vi "disc_PI.vi"(0 "y_ref":dbl, 1 "PISettiings":cluster{"Kp":dbl, "Ti":dbl}, 2 "Ts":dbl, 3 "manual":u16, 4 "u_man":dbl, 5 "y":dbl) -> (14 "u_k":dbl)   [LabVIEW 2019]
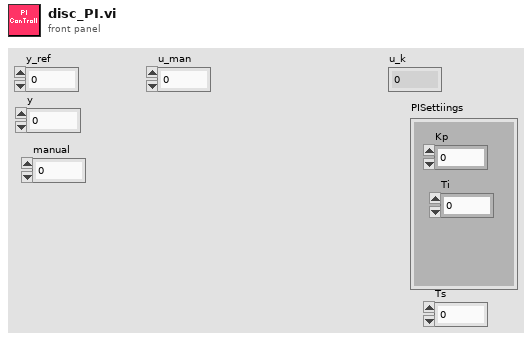
[diagram p1: front panel]
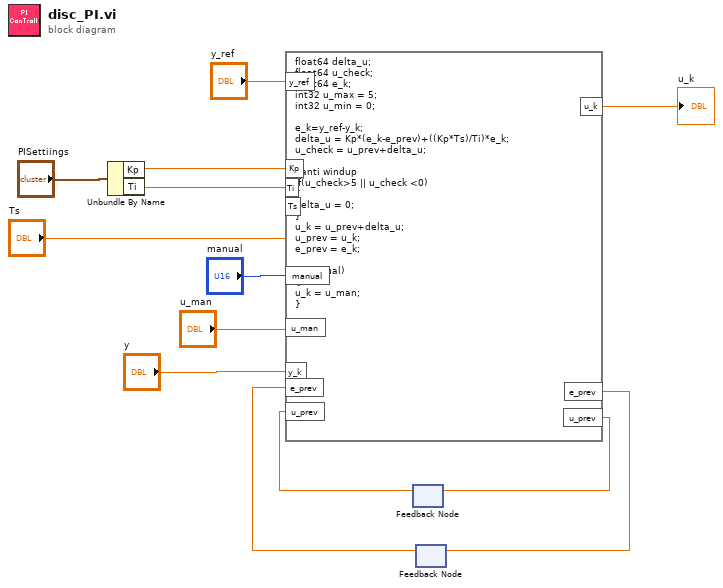
[diagram p0: block diagram]
diagram:
  n1 = Unbundle By Name("PISettiings") -> ("Kp"=w6:dbl, "Ti"=w5:dbl)
  n2 = feedback #1() -> (w8:dbl)  [unwired: 1 in]
  n3 = feedback #2() -> (w2:dbl)  [unwired: 1 in]
  n4 = formula code="float64 delta_u;\nfloat64 u_check;\nfloat64 e_k;\nint32 u_max = 5;\nint32 u_min = 0;\n\ne_k=y_ref-y_k;\ndelta_u = Kp*(e_k-e_prev)+((Kp*Ts)/Ti)*e_k;\nu_check = u_prev+delta_u;\n\n//anti windup\nif(u_check>5 || u_check <0)\n{\ndelta_u = 0;\n}\nu_k = u_prev+delta_u;\nu_prev = u_k;\ne_prev = e_k;\n\nif(manual)\n{\nu_k = u_man;\n}"("y_ref"="y_ref", "y_k"="y", "e_prev"=w2, "Kp"=w6, "Ti"=w5, "Ts"="Ts", "u_prev"=w8, "manual"="manual", "u_man"="u_man") -> ("u_k"=→"u_k":dbl, "u_prev"=w9:dbl, "e_prev"=w3:dbl)
  n5 = feedback-in #1(w9) -> ()
  n6 = feedback-in #2(w3) -> ()
